vi "doAction.vi"(8 "error in (no error)":errorcluster, 10 "ContextData":refnum<class "ContextData.lvclass">, 11 "User State 2 in":refnum<class "Lost.lvclass">) -> (0 "error out":errorcluster, 2 "ContextData Out":refnum<class "ContextData.lvclass">, 3 "User State 2 out":refnum<class "Lost.lvclass">)   [LabVIEW 2019, in "Lost.lvclass"]
uses:
  Lost.lvclass
  ContextData/ContextData.lvclass
  5daf2153-19ab-4107-8d5e-6667ab779e21.vi
  uiControlsMgr/uiControlsMgr.lvclass
  Messages/simonMessages/simonMessages.lvclass
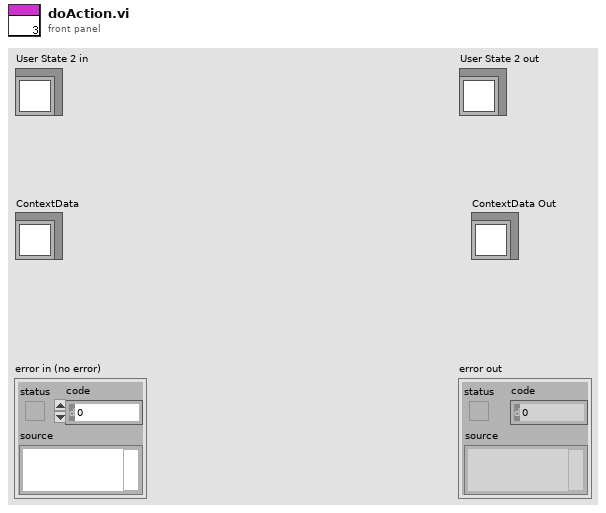
[diagram p1: front panel]
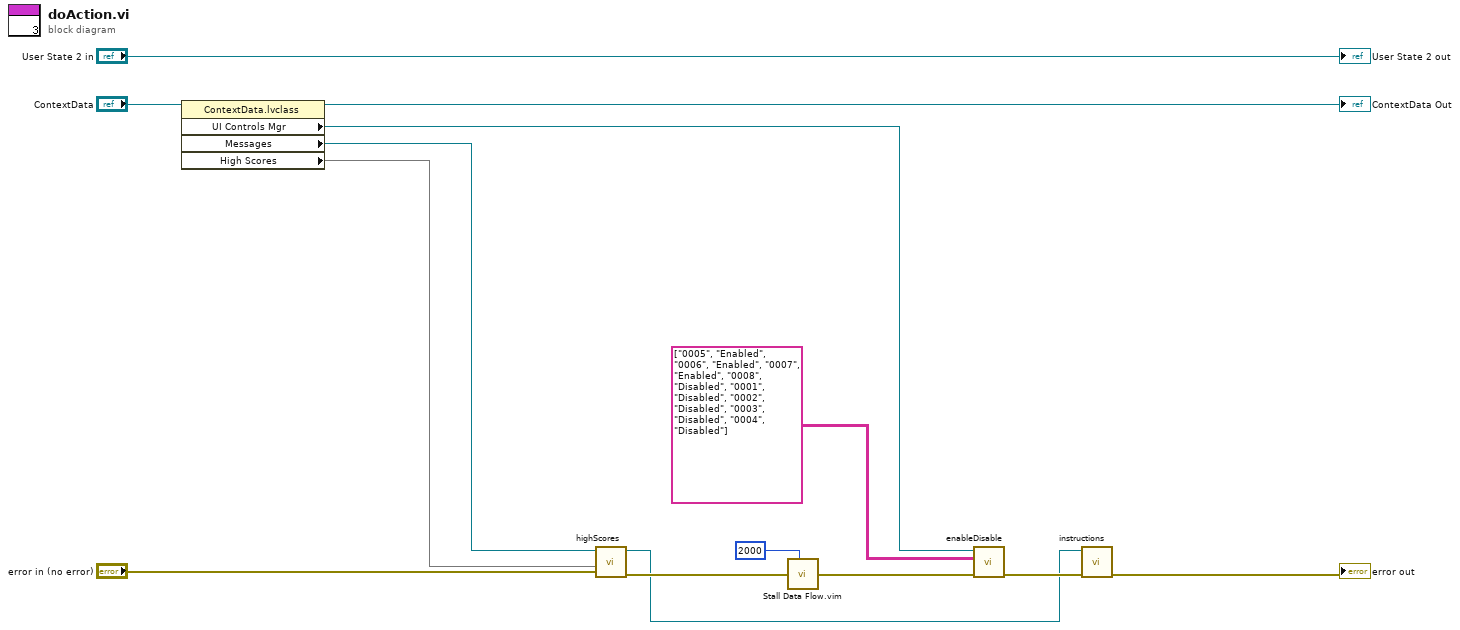
[diagram p0: block diagram]
diagram:
  n1 = property class="ContextData.lvclass"(reference="ContextData") -> (reference out=→"ContextData Out":refnum<class "ContextData.lvclass">, "UI Controls Mgr"=w3:refnum<class "uiControlsMgr.lvclass">, "Messages"=w2:refnum<class "simonMessages.lvclass">, "High Scores"=w1:map{string, i32})  [unwired: 1 in, 1 out]
  n2 = call "highScores.vi"("error in (no error)"="error in (no error)", "High Scores"=w1, "simonMessages in"=w2) -> ("error out"=w11:errorcluster, "simonMessages out"=w4:refnum<class "simonMessages.lvclass">)  [unwired: 7 in]
  n3 = call "Stall Data Flow.vim"("value in"=w11, "milliseconds to wait"=u32 2000) -> ("value out"=w10:errorcluster)  [unwired: 1 out]
  n4 = call "enableDisable.vi"("error in (no error)"=w10, "Controls - Status"=string[][] [["0005", "Enabled"], ["0006", "Enabled"], ["0007", "Enabled"], ["0008", "Disabled"], ["0001", "Disabled"], ["0002", "Disabled"], ["0003", "Disabled"], ["0004", "Disabled"]], "uiControlsMgr in"=w3) -> ("error out"=w8:errorcluster)  [unwired: 7 in, 1 out]
  n5 = call "instructions.vi"("error in (no error)"=w8, "simonMessages in"=w4) -> ("error out"=→"error out":errorcluster)  [unwired: 8 in, 1 out]
  "User State 2 out" <- "User State 2 in"
